vi "지도만들기_TEST.vi"() -> ()   [LabVIEW 2023]
uses:
  <vilib>/httpClient/LabVIEWHTTPClient.lvlib
panel:
  out "new picture 2":picture caption="새 그림"
  in  "WebBrowser":refnum<k7>(container) caption="웹 브라우저"
  in  "Map Format":string(combo)="roadmap"
  in  "Size X":dbl=450.0
  in  "Size Y":dbl=650.0
  in  "Zoom":sgl=16.0 format="%#.1g"
  in  "Logitude":string="129.15510"
  in  "Latitude":string="35.17100"
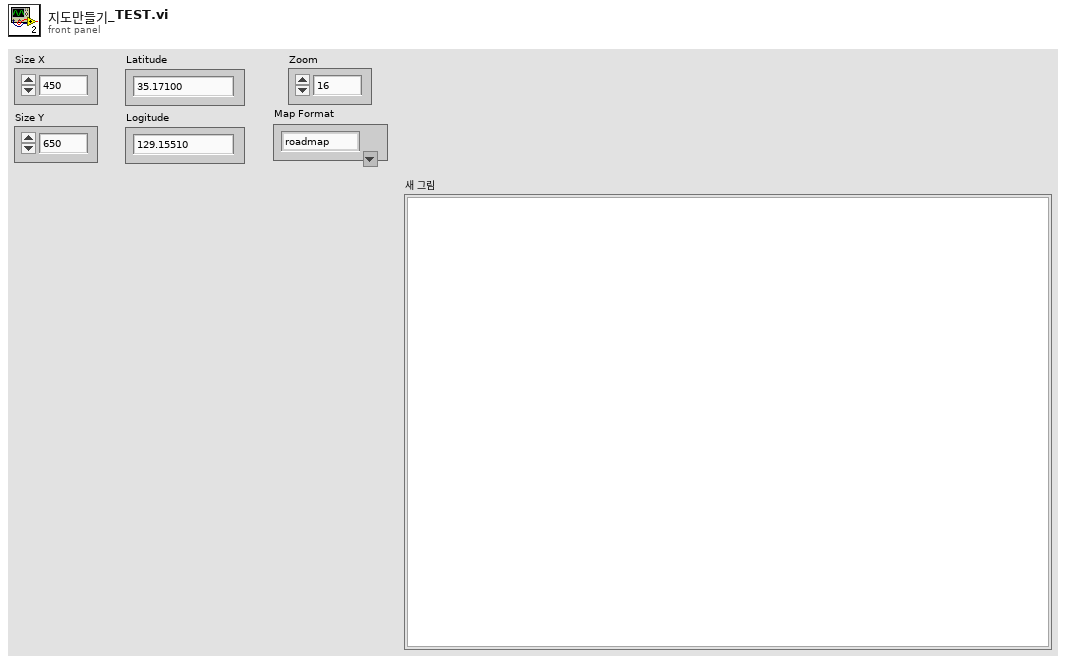
[diagram p1: front panel]
types:
  T1 = cluster{"Width":u16, "Style":enum32{"Solid", "Dash", "Dot", "DashDot", "DashDotDot"}}
  T2 = cluster{"Marker":string, "Path":string, "Markers Coordinates":string[][]}
  T3 = typedef "LabVIEWHTTPClient.lvlib/ClientHandle.ctl" = refnum<k1>
  T4 = typedef "imagedata.ctl" = cluster{"image type":i32, "image depth":i32, "image":u8[], "mask":u8[], "colors":u32[], "Rectangle":cluster{"left":i16, "top":i16, "right":i16, "bottom":i16}}
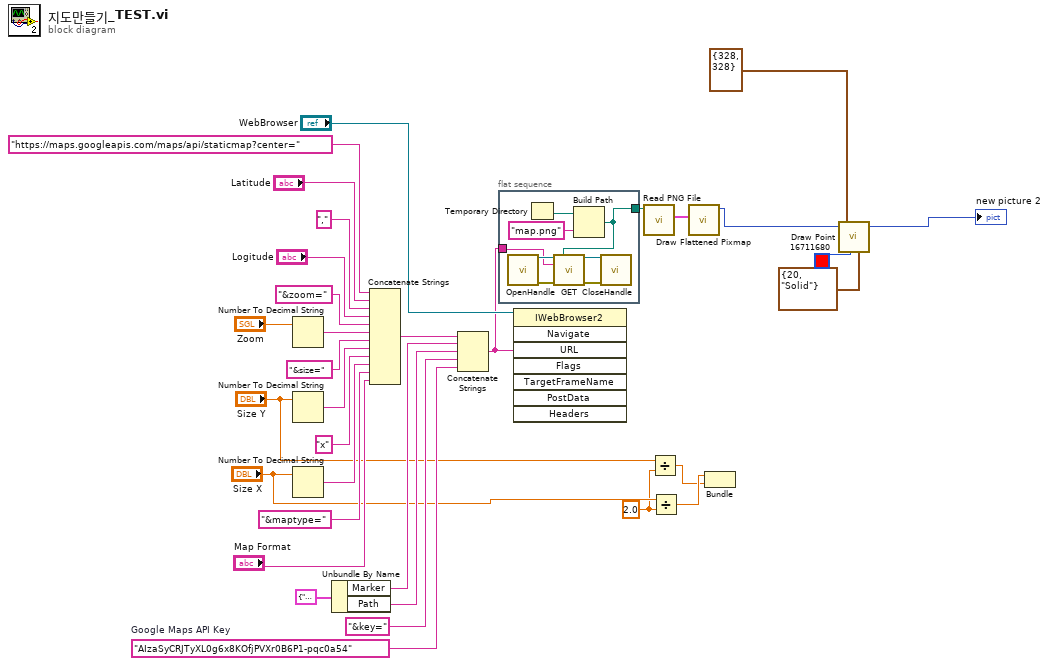
[diagram p0: block diagram]
diagram:
  w8 = 2.0 ("y")
  w15 = "AIzaSyCRJTyXL0g6x8KOfjPVXr0B6P1-pqc0a54"  # Google Maps API Key
  n1 = Number To Decimal String(number="Zoom") -> (decimal integer string=w28:string)  [unwired: 1 in]
  n2 = Number To Decimal String(number="Size Y") -> (decimal integer string=w30:string)  [unwired: 1 in]
  n3 = Number To Decimal String(number="Size X") -> (decimal integer string=w32:string)  [unwired: 1 in]
  n4 = Unbundle By Name(T2 {"Marker"="", "Path"="", "Markers Coordinates"=[]}) -> ("Marker"=w18:string, "Path"=w17:string)
  n5 = Concatenate Strings("https://maps.googleapis.com/maps/api/staticmap?center=" ("URL"), "Latitude", "," ("string"), "Logitude", "&zoom=", w28, "&size=", w30, "x", w32, "&maptype=", "Map Format") -> (w19:string)
  n6 = Concatenate Strings(w19, w18, w17, "&key=" ("string"), w15) -> (w13:string)
  n7 = flat-sequence {
    tunnel: w13 -> [w37]
    tunnel: [w34] -> w12
    frame #0 {
      n8 = call <vilib>:"OpenHandle.vi"() -> ("client handle out"=w41:T3, "error out"=w40:errorcluster)  [unwired: 14 in]
      n9 = Temporary Directory() -> (w35:path)
      n10 = Build Path(base path=w35, name or relative path="map.png") -> (appended path=w34:path)
      n11 = call <vilib>:"GET.vi"("client handle"=w41, "output file"=w34, "url"=w37, "error in (no error)"=w40) -> ("client handle out"=w38:T3, "error out"=w39:errorcluster)  [unwired: 8 in, 2 out]
      n12 = call <vilib>:"CloseHandle.vi"("client handle"=w38, "error in (no error)"=w39) -> ()  [unwired: 13 in, 1 out]
    }
  }
  n13 = invoke class="IWebBrowser2" method="Navigate"(reference="WebBrowser", "URL"=w13) -> ()  [unwired: 6 in, 8 out]
  n14 = call <vilib>:"Read PNG File.vi"("path to PNG file"=w12) -> ("image data"=w11:T4)  [unwired: 8 in, 2 out]
  n15 = Divide(x="Size Y", y=w8) -> (x/y=w5:dbl)
  n16 = Divide(x="Size X", y=w8) -> (x/y=w6:dbl)
  n17 = call <vilib>:"Draw Flattened Pixmap.vi"("image data"=w11) -> ("new picture"=w10:picture)  [unwired: 1 in, 7 out]
  n18 = Bundle(w6, w5) -> ()  [unwired: 1 in, 1 out]
  n19 = call <vilib>:"Draw Point.vi"("picture"=w10, "point(x,y)"=cluster{"x":i16, "y":i16} {"x"=328, "y"=328}, "color(black)"=u32 16711680, "pen"=T1 {"Width"=20, "Style"=enum."Solid"}) -> ("new picture"=→"new picture 2":picture)  [unwired: 5 in]
